vi "Test App Processes Receive all calls.vi"(8 "error in (no error)":errorcluster, 11 "Rig Test In":refnum<class "Application Dev Test.lvclass">) -> (0 "error out":errorcluster, 3 "Rig Test Out":refnum<class "Application Dev Test.lvclass">)   [LabVIEW 2020, in "Application Dev Test.lvclass"]
uses:
  Application Dev Test.lvclass
  C:/Program Files (x86)/National Instruments/LabVIEW 2020/vi.lib/Astemes/LUnit/Test Case.lvclass
  source/Framework Test Suite/Mock Process/Mock Process.lvclass
  C:/Git/astemes-triarc-framework/source/Framework/Process/Process.lvclass
  source/Framework/Process/Process.lvclass/Process.ctl
  source/Framework/Application/Application.lvclass/Application.ctl
  <vilib>/Astemes/LUnit/Test Case.lvclass/Test Case.ctl
  <vilib>/Astemes/LUnit/LUnit Assertion Result.lvclass/LUnit Assertion Result.ctl
  <vilib>/Astemes/LUnit/LUnit Test Case Result.lvclass/LUnit Test Case Result.ctl
  <vilib>/Astemes/LUnit/LUnit Method Result.lvclass/LUnit Method Result.ctl
  source/Framework/Application/Private/Add Process to Map.vi
  source/Framework/Application/Private/Start Idle Processes if Running.vi
  source/Framework/Application/Private/Throw Error If Process Already in App.vi
  source/Framework/Process/Protected/Messaging/Enqueue Message.vi
  source/Framework/Process/Public/Lifecycle/Get Lifecycle State.vi
  source/Framework/Process/Protected/SubVIs/Set Context.vi
  source/Framework/Process/Private/SubVIs/Wait for finish.vi
  source/Framework/Process/Private/SubVIs/Set Lifecycle State.vi
  <vilib>/Astemes/LUnit/Palette/Fail.vi
  <vilib>/Astemes/LUnit/Palette/Pass.vi
  <vilib>/Astemes/LUnit/Set Assertion Type.vi
  source/Framework/Application/Public/Get Process.vi
  source/Framework/Process/Private/SubVIs/Handle Debug Data.vi
  <vilib>/Utility/error.llb/Clear Errors.vi
  source/Framework/Process/Public/Lifecycle/Leave Process Loop.vi
  <vilib>/Astemes/LUnit/Add test result.vi
  <vilib>/Astemes/LUnit/LUnit Write Passed.vi
  <vilib>/Astemes/LUnit/LUnit Write Message.vi
  <vilib>/Astemes/LUnit/LUnit Write Description.vi
  <vilib>/Astemes/LUnit/LUnit Write Assertion Type.vi
  source/Framework/Application/Private/Retrieve Process from App.vi
  source/Framework/Application/Private/Parse Process Name.vi
  source/Framework/Application/Private/Get Process from Map.vi
  source/Framework/Logging/Log Debug.vi
  <vilib>/AdvancedString/1D String Array to Delimited String.vi
  <vilib>/Utility/High Resolution Relative Seconds.vi
  <vilib>/Astemes/LUnit/LUnit Record Assertion Result.vi
  source/Framework/Process/Protected/Messaging/Request Message.vi
  <vilib>/AdvancedString/Delimited String to 1D String Array.vi
  <vilib>/Astemes/LUnit/LUnit Aggregate Assertion Results.vi
  source/Framework/Process/Private/SubVIs/Enqueue Request Message.vi
  <vilib>/Astemes/LUnit/Assertion Result/LUnit Read Status.vi
  <vilib>/Astemes/LUnit/LUnit Read Message.vi
  <vilib>/Astemes/LUnit/LUnit Read Description.vi
  <vilib>/Astemes/LUnit/Method Result/LUnit Merge Status.vi
  <vilib>/Astemes/LUnit/LUnit Concatenate result strings.vi
  source/Framework/Application/Application.lvclass
  <vilib>/Utility/error.llb/Error Cluster From Error Code.vi
  source/Framework/Process/Public/Read Name.vi
  source/Framework/Process/Private/SubVIs/Wait for Response Message.vi
  source/Framework/Process/Process.lvclass
  <vilib>/Astemes/LUnit/LUnit Assertion Result.lvclass
  Application Dev Test.lvclass/Application Dev Test.ctl
  <vilib>/Astemes/LUnit/Test Case.lvclass
panel:
  out "Messages":string[](array[string])
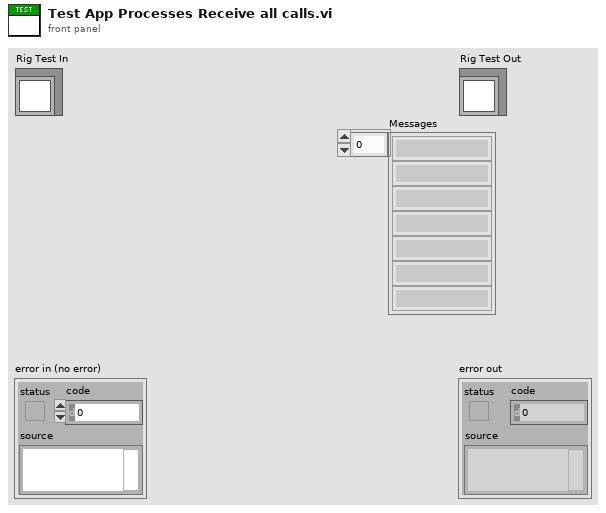
[diagram p1: front panel]
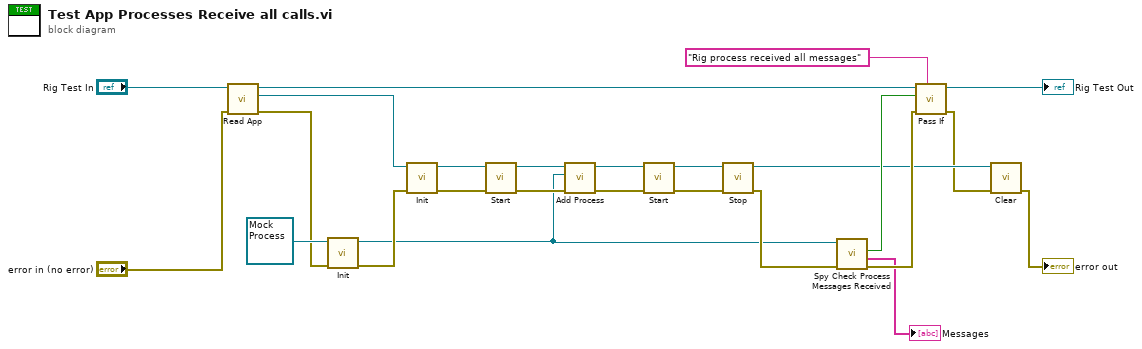
[diagram p0: block diagram]
diagram:
  n1 = call "Read App.vi"("error in (no error)"="error in (no error)", "Application Test In"="Rig Test In") -> ("error out"=w8:errorcluster, "App out"=w9:refnum<class "Application.lvclass">, "Application Test Out"=w24:refnum<class "Application Dev Test.lvclass">)  [unwired: 7 in]
  n2 = call-dynamic "Init.vi"("error in (no error)"=w8, "Mock Process In"=refnum<class "Mock Process.lvclass"> refnum ("Mock Classes.lvlib:Mock Process.lvclass")) -> ("error out"=w14:errorcluster, "Mock Process Out"=w10:refnum<class "Mock Process.lvclass">)  [unwired: 8 in]
  n3 = call-dynamic "Init.vi"("error in (no error)"=w14, "Process In"=w9) -> ("error out"=w21:errorcluster, "Process Out"=w22:refnum<class "Application.lvclass">)  [unwired: 8 in]
  n4 = call "Start.vi"("error in (no error)"=w21, "Process In"=w22) -> ("error out"=w20:errorcluster, "Process Out"=w16:refnum<class "Application.lvclass">)  [unwired: 7 in, 1 out]
  n5 = call "Add Process.vi"("error in (no error)"=w20, "Process"=w10, "Application In"=w16) -> ("error out"=w7:errorcluster, "Application Out"=w6:refnum<class "Application.lvclass">)  [unwired: 7 in]
  n6 = call "Start.vi"("error in (no error)"=w7, "Process In"=w6) -> ("error out"=w18:errorcluster, "Process Out"=w19:refnum<class "Application.lvclass">)  [unwired: 7 in, 1 out]
  n7 = call "Stop.vi"("error in (no error)"=w18, "Process In"=w19) -> ("error out"=w17:errorcluster, "Process Out"=w3:refnum<class "Application.lvclass">)  [unwired: 7 in, 1 out]
  n8 = call "Spy Check Process Messages Received.vi"("error in (no error)"=w17, "Mock Process In"=w10) -> ("error out"=w5:errorcluster, "Messages"=→"Messages":string[], "Messages received?"=w12:bool)  [unwired: 6 in, 1 out]
  n9 = call <vilib>:"Pass If.vi"("Description"="Rig process received all messages", "error in (no error)"=w5, "Pass?"=w12, "LUnit Test Case In"=w24) -> ("error out"=w2:errorcluster, "LUnit Test Case Out"=→"Rig Test Out":refnum<class "Application Dev Test.lvclass">)  [unwired: 6 in]
  n10 = call-dynamic "Clear.vi"("error in (no error)"=w2, "Application In"=w3) -> ("error out"=→"error out":errorcluster)  [unwired: 9 in]
